vi "serenial.io-ase tidy unused files.vi"() -> ()   [LabVIEW 2020]
uses:
  39fbe9b6-994c-4b93-b5b5-6e6fc33ceced.vi
panel:
  out "#Files to Move to Trash":i32
  out "Files That Could Not Be Moved":path[](array[path])
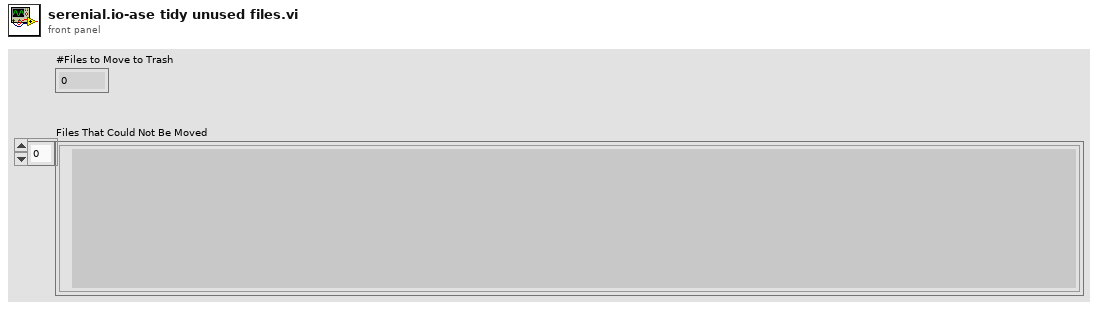
[diagram p1: front panel]
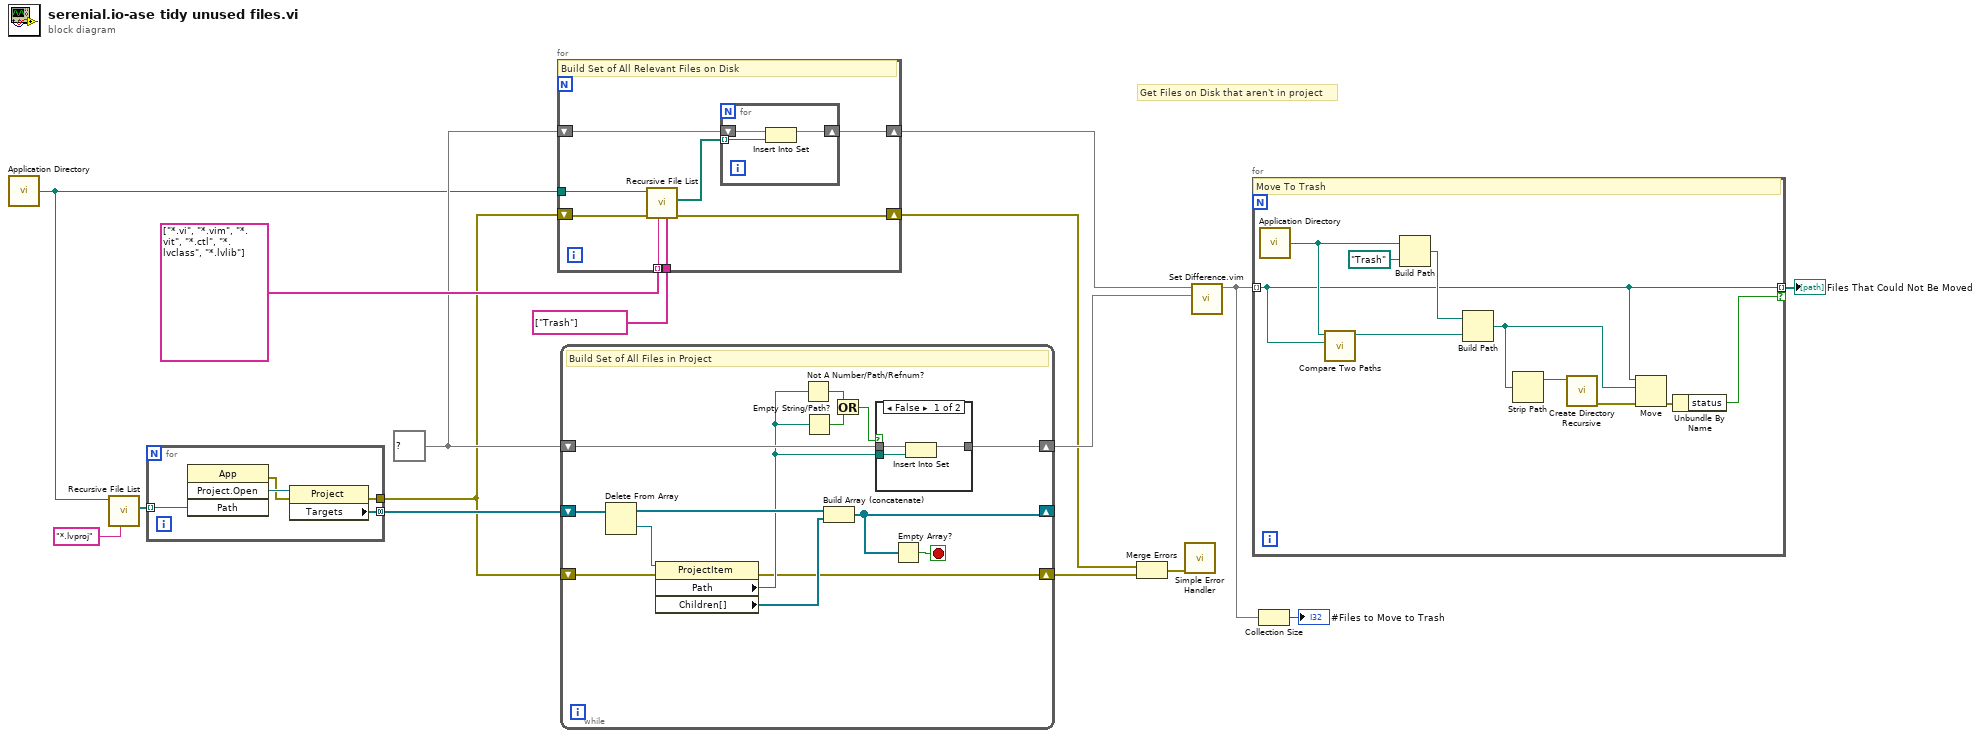
[diagram p0: block diagram]
diagram:
  w14 = set{path} {} ("Size: 0")
  # "Get Files on Disk that aren't in project"
  n1 = call <vilib>:"Application Directory.vi"() -> ("Application Directory"=w4:path)
  n2 = call <vilib>:"Recursive File List.vi"("pattern"="*.lvproj", "Folder Path"=w4) -> ("All Files in Dir"=w2:path[])  [unwired: 5 in, 4 out]
  n3 = for {
    tunnel: [w19] -> w16 mode=concatenating
    tunnel: [w18] -> w10
    tunnel: w2 -> [w17] mode=indexing
    n4 = invoke class="App" method="Project.Open"("Path"=w17) -> (error out=w20:errorcluster, "Project:Open"=w21:refnum<vi>)  [unwired: 3 in, 2 out]
    n5 = property class="Project"(reference=w21, error in=w20) -> (error out=w18:errorcluster, "Targets"=w19:refnum<vi>[])  [unwired: 1 out]
  }
  n6 = for {
    tunnel: w4 -> [w29]
    tunnel: string[] ["*.vi", "*.vim", "*.vit", "*.ctl", "*.lvclass", "*.lvlib"] -> [w27] mode=indexing
    shift-right: [w26] -> w8
    shift-left: w10 -> [w28]
    shift-right: [w23] -> w13
    shift-left: w14 -> [w24]
    tunnel: string[] ["Trash"] ("Folders to Exclude") -> [w22]
    # "Build Set of All Relevant Files on Disk"
    n7 = call <vilib>:"Recursive File List.vi"("Folders to Exclude"=w22, "pattern"=w27, "error in (no error)"=w28, "Folder Path"=w29) -> ("error out"=w26:errorcluster, "All Files in Dir"=w25:path[])  [unwired: 3 in, 3 out]
    n8 = for {
      tunnel: w25 -> [w31] mode=indexing
      shift-right: [w30] -> w23
      shift-left: w24 -> [w32]
      n9 = Insert Into Set(10:w31, 11:w32) -> (3:w30:set{path})  [unwired: 1 out]
    }
  }
  n10 = while {
    shift-right: [w46] -> w12
    shift-left: w14 -> [w45]
    shift-right: [w40] -> _
    shift-left: w16 -> [w44]
    shift-right: [w33] -> w9
    shift-left: w10 -> [w34]
    stop <- w39 stop-if-true
    # "Build Set of All Files in Project"
    n11 = Delete From Array(array=w44) -> (deleted portion=w43:refnum<vi>, array with subset deleted=w42:refnum<vi>[])  [unwired: 2 in]
    n12 = property class="ProjectItem"(reference=w43, error in=w34) -> (error out=w33:errorcluster, "Path"=w37:path, "Children[]"=w41:refnum<vi>[])  [unwired: 1 out]
    n13 = Not A Number/Path/Refnum?(number/path/refnum=w37) -> (NaN/Path/Refnum?=w38:bool)
    n14 = Empty String/Path?(string/path=w37) -> (empty?=w35:bool)
    n15 = Build Array (concatenate)(w42, w41) -> (w40:refnum<vi>[])
    n16 = Or(x=w38, y=w35) -> (x .or. y?=w36:bool)
    n17 = case shown="False" w36 {
      tunnel: w37 -> [w49 _]
      tunnel: [w48 w50] -> w46
      tunnel: w45 -> [w47 w50]
      frame False {
        n18 = Insert Into Set(10:w49, 11:w47) -> (3:w48:set{path})  [unwired: 1 out]
      }
      frame True {
      }
    }
    n19 = Empty Array?(array=w40) -> (empty?=w39:bool)
  }
  n20 = Merge Errors(w8, w9) -> (w7:errorcluster)
  n21 = call <vilib>:"Simple Error Handler.vi"("error in (no error)"=w7) -> ()  [unwired: 4 in, 5 out]
  n22 = call "Set Difference.vim"("set 2"=w12, "set 1"=w13) -> ("difference"=w6:set{path})  [unwired: 9 in]
  n23 = for {
    tunnel: w6 -> [w53] mode=indexing
    tunnel: [w53] -> w11 mode=indexing if=w51
    # "Move To Trash"
    n24 = call <vilib>:"Application Directory.vi"() -> ("Application Directory"=w60:path)
    n25 = call <vilib>:"Compare Two Paths.vi"("Path 2"=w53, "Path 1"=w60) -> ("Relative Path from 1 to 2"=w57:path)  [unwired: 6 in, 3 out]
    n26 = Build Path(base path=w60, name or relative path=path "Trash") -> (appended path=w58:path)
    n27 = Build Path(base path=w58, name or relative path=w57) -> (appended path=w54:path)
    n28 = Strip Path(path=w54) -> (stripped path=w56:path)  [unwired: 1 out]
    n29 = call <vilib>:"Create Directory Recursive.vi"("directory"=w56) -> ("error out"=w55:errorcluster)  [unwired: 4 in, 2 out]
    n30 = Move(source path=w53, error in=w55, 10:w54) -> (error out=w52:errorcluster)  [unwired: 2 in, 2 out]
    n31 = Unbundle By Name(w52) -> ("status"=w51:bool)
  }
  "Files That Could Not Be Moved" <- w11
  n32 = Collection Size(1:w6) -> (0:→"#Files to Move to Trash":i32)
